vi "hmi_initialize.vi"(4 "dialog_type":T3=enum."one_button", 6 "configuration":T2={"dialog_text"="", "boolean_text_1"="", "boolean_text_2"="", "boolean_text_3"="", "inner_color"=16711680, "outer_color"=6618880, "wait_s"=nan, "error_status"=FALSE, "error_source"="", "error_details"="", "string []"=[], "custom_entry"=FALSE}, 7 "references":T1, 8 "error in (no error)":errorcluster) -> (0 "error out":errorcluster)   [LabVIEW 2015, in "lv-dialog-interfaces.lvlib"]
uses:
  lv-dialog-interfaces.lvlib
  _controls/dialog_type.ctl
  _controls/configuration.ctl
  _controls/hmi_references.ctl
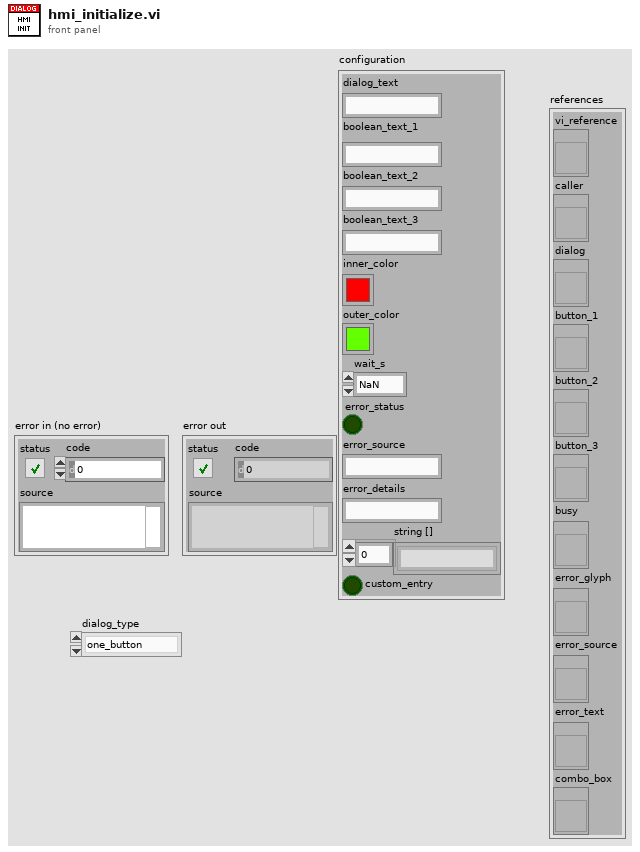
[diagram p1: front panel]
types:
  T1 = typedef "lv-dialog-interfaces.lvlib/hmi_references.ctl" = cluster{"vi_reference":refnum<vi>, "caller":refnum<vi>, "dialog":refnum<vi>, "button_1":refnum<vi>, "button_2":refnum<vi>, "button_3":refnum<vi>, "busy":refnum<vi>, "error_glyph":refnum<vi>, "error_source":refnum<vi>, "error_text":refnum<vi>, "combo_box":refnum<vi>}
  T2 = typedef "lv-dialog-interfaces.lvlib/configuration.ctl" = cluster{"dialog_text":string, "boolean_text_1":string, "boolean_text_2":string, "boolean_text_3":string, "inner_color":u32, "outer_color":u32, "wait_s":dbl, "error_status":bool, "error_source":string, "error_details":string, "string []":string[], "custom_entry":bool}
  T3 = typedef "lv-dialog-interfaces.lvlib/dialog_type.ctl" = enum16{"null", "one_button", "two_button", "three_button", "confirmation", "busy_wait", "error", "busy_wait_embed", "combo_box", "data_entry_string", "data_entry_numeric"}
  T4 = cluster{"max_height":i16, "max_width":i16, "control_height":i16, "control_width":i16}
  T5 = enum8{"Enabled", "Disabled", "Disabled and Grayed Out"}
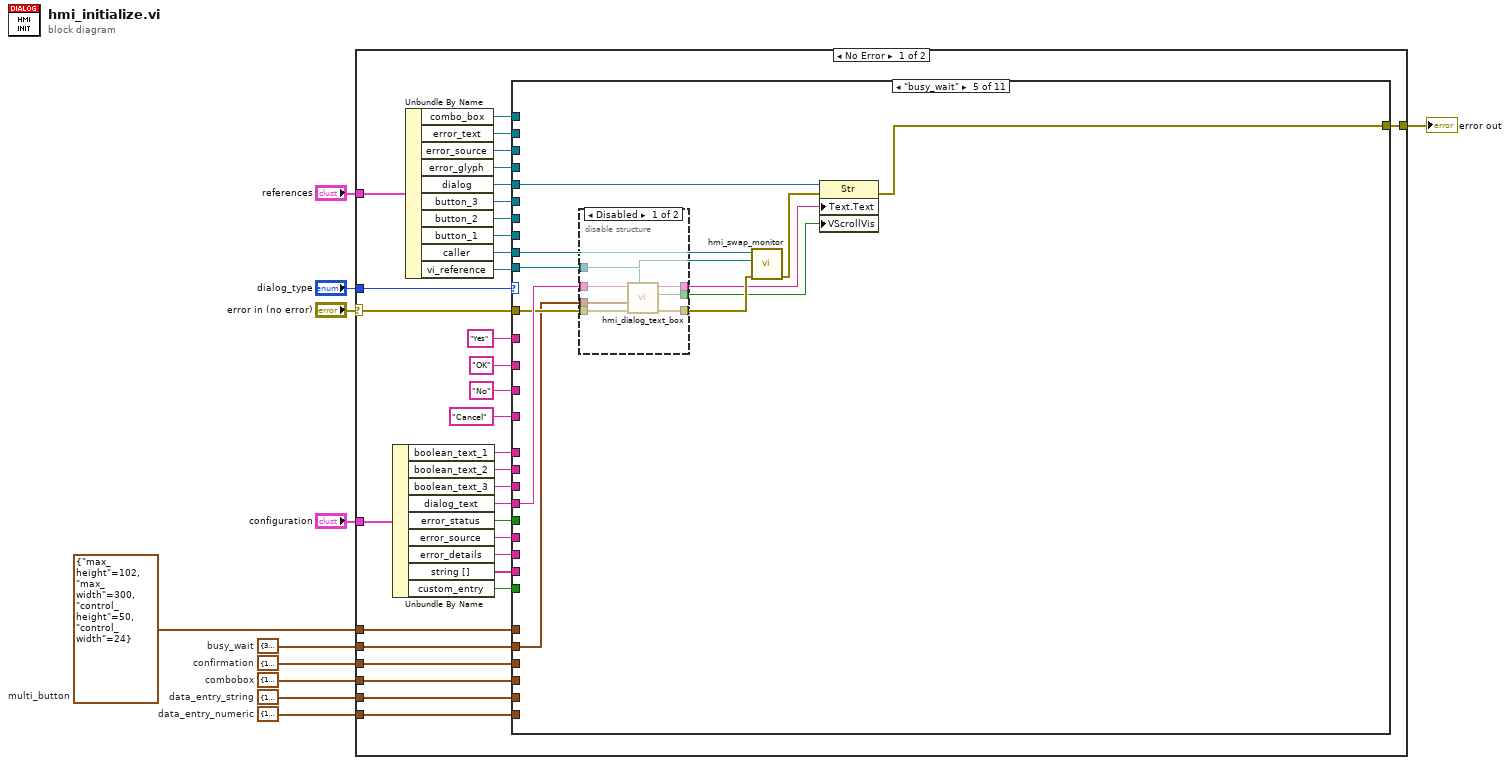
[diagram p0: block diagram]
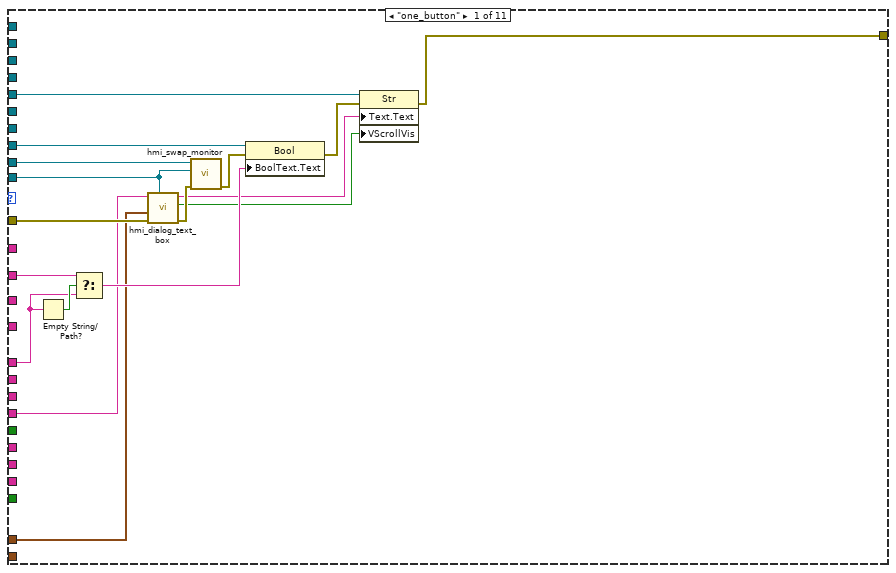
[diagram p2: hidden frame]
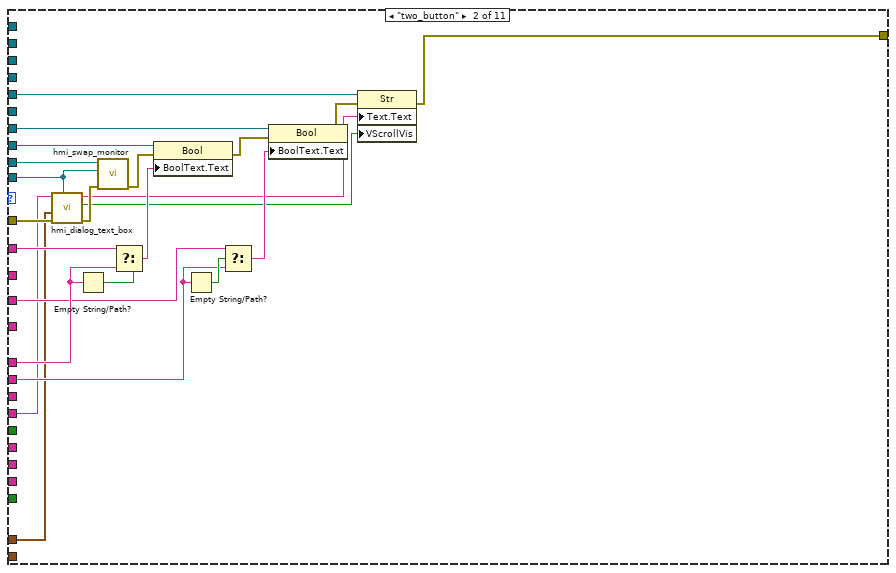
[diagram p3: hidden frame]
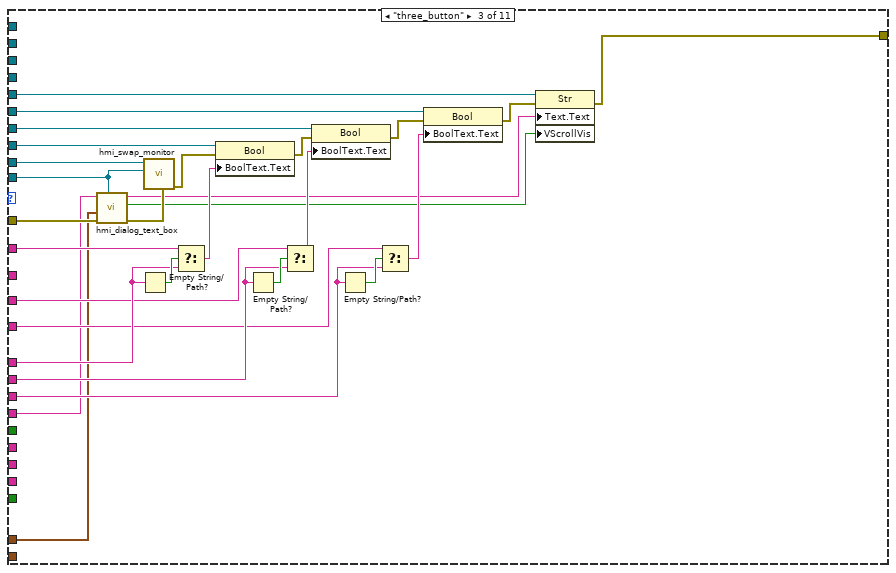
[diagram p4: hidden frame]
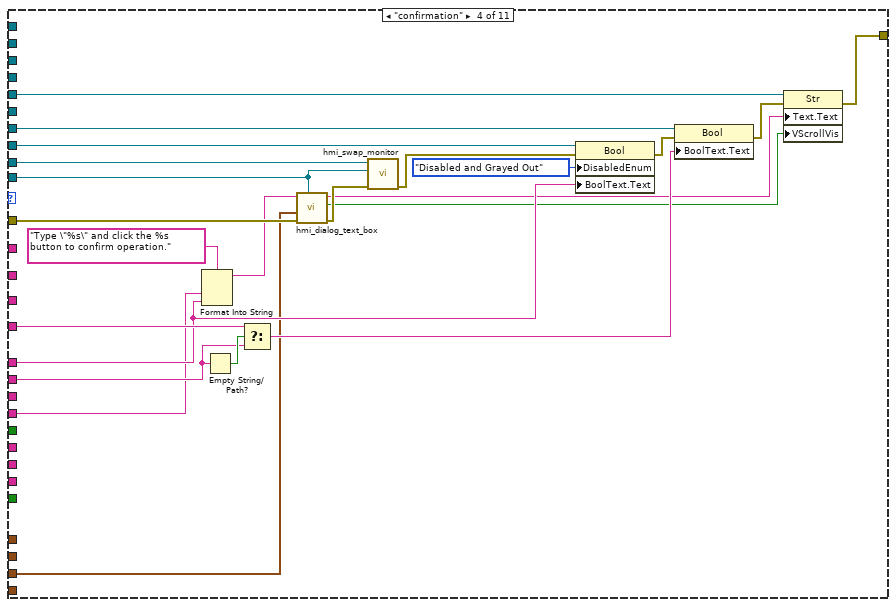
[diagram p5: hidden frame]
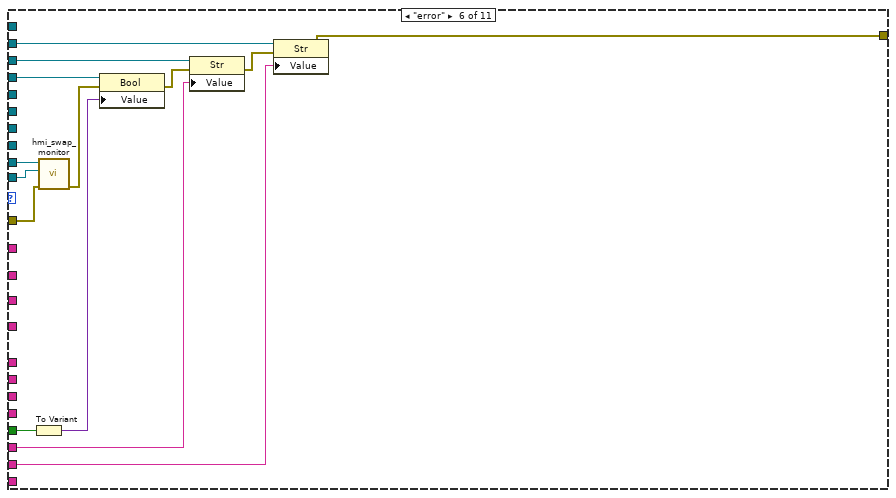
[diagram p7: hidden frame]
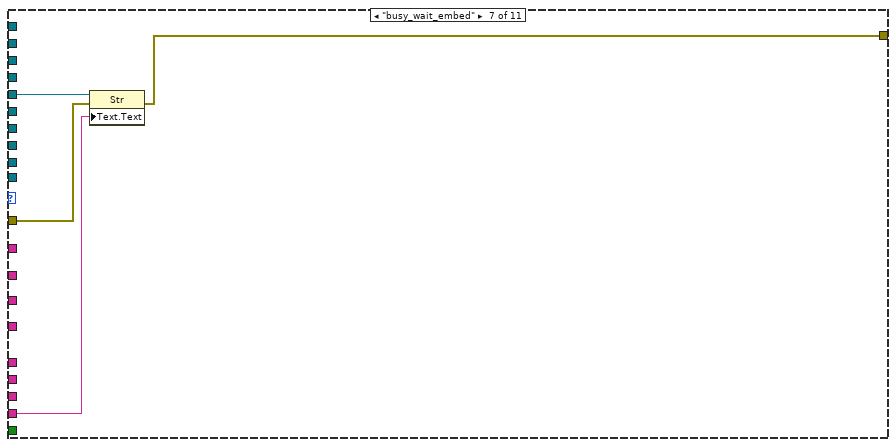
[diagram p8: hidden frame]
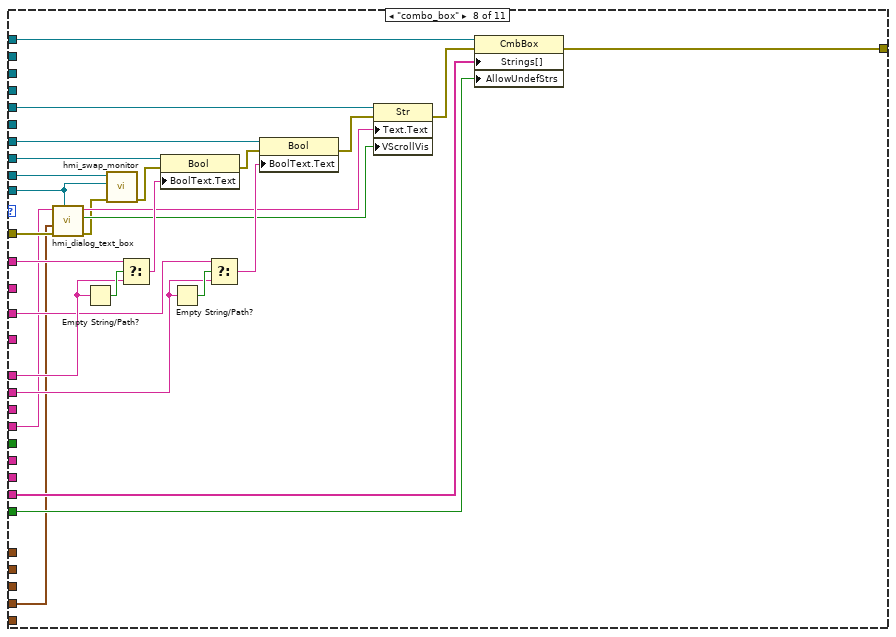
[diagram p9: hidden frame]
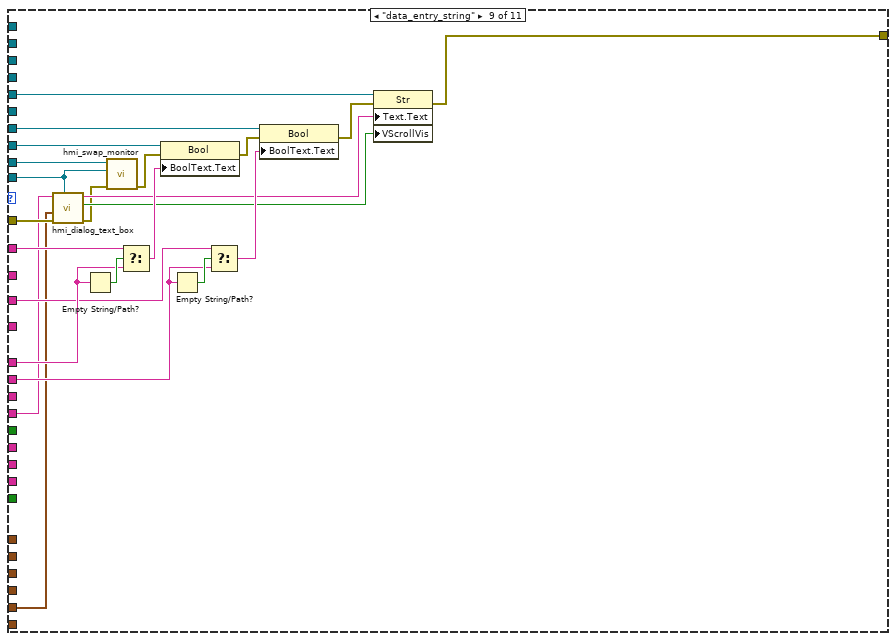
[diagram p10: hidden frame]
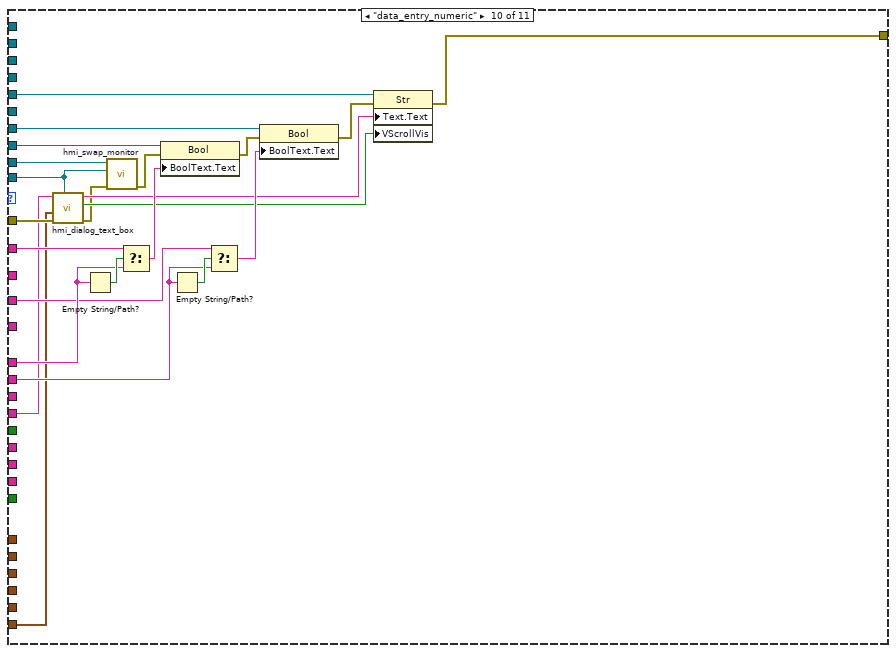
[diagram p11: hidden frame]
diagram:
  w1 = T4 {"max_height"=102, "max_width"=300, "control_height"=50, "control_width"=24}  # data_entry_numeric
  w2 = T4 {"max_height"=102, "max_width"=300, "control_height"=50, "control_width"=24}  # data_entry_string
  w5 = T4 {"max_height"=300, "max_width"=175, "control_height"=175, "control_width"=24}  # busy_wait
  w3 = T4 {"max_height"=102, "max_width"=300, "control_height"=50, "control_width"=24}  # combobox
  w4 = T4 {"max_height"=102, "max_width"=300, "control_height"=50, "control_width"=24}  # confirmation
  w6 = T4 {"max_height"=102, "max_width"=300, "control_height"=50, "control_width"=24}  # multi_button
  n1 = case shown="No Error" "error in (no error)" {
    selector: "error in (no error)" -> [w28 w250]
    tunnel: [w44 w250] -> w10
    tunnel: "dialog_type" -> [w45 _]
    tunnel: "configuration" -> [w39 _]
    tunnel: "references" -> [w43 _]
    tunnel: w6 -> [w17 _]
    tunnel: w5 -> [w16 _]
    tunnel: w4 -> [w15 _]
    tunnel: w3 -> [w14 _]
    tunnel: w2 -> [w13 _]
    tunnel: w1 -> [w12 _]
    frame No Error {
      n2 = Unbundle By Name(w39) -> ("boolean_text_1"=w38:string, "boolean_text_2"=w37:string, "boolean_text_3"=w36:string, "dialog_text"=w35:string, "error_status"=w27:bool, "error_source"=w26:string, "error_details"=w25:string, "string []"=w19:string[], "custom_entry"=w18:bool)
      n3 = Unbundle By Name(w43) -> ("combo_box"=w20:refnum<vi>, "error_text"=w24:refnum<vi>, "error_source"=w23:refnum<vi>, "error_glyph"=w22:refnum<vi>, "dialog"=w42:refnum<vi>, "button_3"=w41:refnum<vi>, "button_2"=w40:refnum<vi>, "button_1"=w34:refnum<vi>, "caller"=w21:refnum<vi>, "vi_reference"=w29:refnum<vi>)
      n4 = case shown="\"busy_wait\"" w45 {
        tunnel: w28 -> [w55 w70 w91 w121 w146 w162 w172 w185 w211 w234 w249]
        tunnel: [w52 w63 w93 w123 w140 w163 w173 w188 w204 w227 w249] -> w44
        tunnel: w42 -> [w53 w67 w94 w133 w141 _ w174 w182 w208 w231 _]
        tunnel: w41 -> [_ _ w114 _ _ _ _ _ _ _ _]
        tunnel: w40 -> [_ w85 w113 w137 _ _ _ w202 w225 w248 _]
        tunnel: w38 -> [w61 w83 w111 w127 _ _ _ w200 w223 w246 _]
        tunnel: w37 -> [_ w81 w108 w135 _ _ _ w198 w221 w244 _]
        tunnel: w36 -> [_ _ w107 _ _ _ _ _ _ _ _]
        tunnel: w35 -> [w47 w69 w89 w117 w147 _ w175 w184 w210 w233 _]
        tunnel: w34 -> [w60 w78 w103 w134 _ _ _ w195 w218 w241 _]
        tunnel: "OK" -> [w58 _ _ _ _ _ _ _ _ _ _]
        tunnel: "Cancel" -> [_ _ w104 w130 _ _ _ _ _ _ _]
        tunnel: "Yes" -> [_ w80 w106 _ _ _ _ w197 w220 w243 _]
        tunnel: "No" -> [_ w79 w105 _ _ _ _ w196 w219 w242 _]
        tunnel: w27 -> [_ _ _ _ _ w168 _ _ _ _ _]
        tunnel: w26 -> [_ _ _ _ _ w167 _ _ _ _ _]
        tunnel: w25 -> [_ _ _ _ _ w166 _ _ _ _ _]
        tunnel: w24 -> [_ _ _ _ _ w169 _ _ _ _ _]
        tunnel: w23 -> [_ _ _ _ _ w170 _ _ _ _ _]
        tunnel: w22 -> [_ _ _ _ _ w171 _ _ _ _ _]
        tunnel: w21 -> [w57 w74 w97 w124 w148 w160 _ w191 w214 w237 _]
        tunnel: w29 -> [w51 w71 w90 w122 w139 w159 _ w186 w212 w235 _]
        tunnel: w20 -> [_ _ _ _ _ _ _ w189 _ _ _]
        tunnel: w19 -> [_ _ _ _ _ _ _ w187 _ _ _]
        tunnel: w17 -> [w46 w68 w87 _ _ _ _ _ _ _ _]
        tunnel: w18 -> [_ _ _ _ _ _ _ w177 _ _ _]
        tunnel: w16 -> [_ _ _ _ w138 _ _ _ _ _ _]
        tunnel: w15 -> [_ _ _ w115 _ _ _ _ _ _ _]
        tunnel: w14 -> [_ _ _ _ _ _ _ w176 _ _ _]
        tunnel: w13 -> [_ _ _ _ _ _ _ _ w203 _ _]
        tunnel: w12 -> [_ _ _ _ _ _ _ _ _ w226 _]
        frame "one_button" {
          n5 = Empty String/Path?(string/path=w61) -> (empty?=w62:bool)
          n6 = Select(t=w58, s=w62, f=w61) -> (s? t:f=w50:string)
          n7 = call "hmi_dialog_text_box.vi"("vi_reference"=w51, "error in (no error)"=w55, "vi_maximums"=w46, "dialog_text in"=w47) -> ("error out"=w54:errorcluster, "enable_scrollbar"=w48:bool, "dialog_text out"=w49:string)  [unwired: 5 in]
          n8 = call "hmi_swap_monitor.vi"("error in (no error)"=w54, "callee_vi_refnum"=w51, "caller_vi_refnum"=w57) -> ("error out"=w56:errorcluster)  [unwired: 8 in]
          n9 = property class="Bool"(reference=w60, error in=w56, "BoolText.Text"=w50) -> (error out=w59:errorcluster)  [unwired: 1 out]
          n10 = property class="Str"(reference=w53, error in=w59, "Text.Text"=w49, "VScrollVis"=w48) -> (error out=w52:errorcluster)  [unwired: 1 out]
        }
        frame "two_button" {
          n11 = call "hmi_dialog_text_box.vi"("vi_reference"=w71, "error in (no error)"=w70, "vi_maximums"=w68, "dialog_text in"=w69) -> ("error out"=w72:errorcluster, "enable_scrollbar"=w65:bool, "dialog_text out"=w66:string)  [unwired: 5 in]
          n12 = Empty String/Path?(string/path=w83) -> (empty?=w84:bool)
          n13 = call "hmi_swap_monitor.vi"("error in (no error)"=w72, "callee_vi_refnum"=w71, "caller_vi_refnum"=w74) -> ("error out"=w73:errorcluster)  [unwired: 8 in]
          n14 = Select(t=w80, s=w84, f=w83) -> (s? t:f=w77:string)
          n15 = property class="Bool"(reference=w78, error in=w73, "BoolText.Text"=w77) -> (error out=w75:errorcluster)  [unwired: 1 out]
          n16 = Empty String/Path?(string/path=w81) -> (empty?=w82:bool)
          n17 = Select(t=w79, s=w82, f=w81) -> (s? t:f=w76:string)
          n18 = property class="Bool"(reference=w85, error in=w75, "BoolText.Text"=w76) -> (error out=w64:errorcluster)  [unwired: 1 out]
          n19 = property class="Str"(reference=w67, error in=w64, "Text.Text"=w66, "VScrollVis"=w65) -> (error out=w63:errorcluster)  [unwired: 1 out]
        }
        frame "three_button" {
          n20 = call "hmi_dialog_text_box.vi"("vi_reference"=w90, "error in (no error)"=w91, "vi_maximums"=w87, "dialog_text in"=w89) -> ("error out"=w92:errorcluster, "enable_scrollbar"=w86:bool, "dialog_text out"=w88:string)  [unwired: 5 in]
          n21 = Empty String/Path?(string/path=w111) -> (empty?=w112:bool)
          n22 = call "hmi_swap_monitor.vi"("error in (no error)"=w92, "callee_vi_refnum"=w90, "caller_vi_refnum"=w97) -> ("error out"=w96:errorcluster)  [unwired: 8 in]
          n23 = Select(t=w106, s=w112, f=w111) -> (s? t:f=w102:string)
          n24 = property class="Bool"(reference=w103, error in=w96, "BoolText.Text"=w102) -> (error out=w99:errorcluster)  [unwired: 1 out]
          n25 = Empty String/Path?(string/path=w108) -> (empty?=w110:bool)
          n26 = Select(t=w105, s=w110, f=w108) -> (s? t:f=w101:string)
          n27 = property class="Bool"(reference=w113, error in=w99, "BoolText.Text"=w101) -> (error out=w98:errorcluster)  [unwired: 1 out]
          n28 = Empty String/Path?(string/path=w107) -> (empty?=w109:bool)
          n29 = Select(t=w104, s=w109, f=w107) -> (s? t:f=w100:string)
          n30 = property class="Bool"(reference=w114, error in=w98, "BoolText.Text"=w100) -> (error out=w95:errorcluster)  [unwired: 1 out]
          n31 = property class="Str"(reference=w94, error in=w95, "Text.Text"=w88, "VScrollVis"=w86) -> (error out=w93:errorcluster)  [unwired: 1 out]
        }
        frame "confirmation" {
          n32 = Format Into String(format string="Type \"%s\" and click the %s button to confirm operation.", w117, w127) -> (resulting string=w116:string)  [unwired: 2 in, 1 out]
          n33 = Empty String/Path?(string/path=w135) -> (empty?=w136:bool)
          n34 = Select(t=w130, s=w136, f=w135) -> (s? t:f=w132:string)
          n35 = call "hmi_dialog_text_box.vi"("vi_reference"=w122, "error in (no error)"=w121, "vi_maximums"=w115, "dialog_text in"=w116) -> ("error out"=w120:errorcluster, "enable_scrollbar"=w119:bool, "dialog_text out"=w118:string)  [unwired: 5 in]
          n36 = call "hmi_swap_monitor.vi"("error in (no error)"=w120, "callee_vi_refnum"=w122, "caller_vi_refnum"=w124) -> ("error out"=w125:errorcluster)  [unwired: 8 in]
          n37 = property class="Bool"(reference=w134, error in=w125, "DisabledEnum"=T5."Disabled and Grayed Out" ("Disabled"), "BoolText.Text"=w127) -> (error out=w131:errorcluster)  [unwired: 1 out]
          n38 = property class="Bool"(reference=w137, error in=w131, "BoolText.Text"=w132) -> (error out=w129:errorcluster)  [unwired: 1 out]
          n39 = property class="Str"(reference=w133, error in=w129, "Text.Text"=w118, "VScrollVis"=w119) -> (error out=w123:errorcluster)  [unwired: 1 out]
        }
        frame "busy_wait" {
          n40 = disable-structure shown="Disabled" {
            disable-tunnel: w147 -> [w155 w157]
            disable-tunnel: w146 -> [w154 w156]
            disable-tunnel: [w153 w156] -> w145
            disable-tunnel: [w152 w157] -> w144
            disable-tunnel: [w151 _] -> w143
            disable-tunnel: w139 -> [w150 _]
            disable-tunnel: w138 -> [w149 _]
            frame Disabled {
              n41 = call "hmi_dialog_text_box.vi"("vi_reference"=w150, "error in (no error)"=w154, "vi_maximums"=w149, "dialog_text in"=w155) -> ("error out"=w153:errorcluster, "enable_scrollbar"=w151:bool, "dialog_text out"=w152:string)  [unwired: 5 in]
            }
            frame Enabled {
            }
          }
          n42 = call "hmi_swap_monitor.vi"("error in (no error)"=w145, "callee_vi_refnum"=w139, "caller_vi_refnum"=w148) -> ("error out"=w142:errorcluster)  [unwired: 8 in]
          n43 = property class="Str"(reference=w141, error in=w142, "Text.Text"=w144, "VScrollVis"=w143) -> (error out=w140:errorcluster)  [unwired: 1 out]
        }
        frame "error" {
          n44 = To Variant(anything=w168) -> (Variant=w158:variant)
          n45 = call "hmi_swap_monitor.vi"("error in (no error)"=w162, "callee_vi_refnum"=w159, "caller_vi_refnum"=w160) -> ("error out"=w161:errorcluster)  [unwired: 8 in]
          n46 = property class="Bool"(reference=w171, error in=w161, "Value"=w158) -> (error out=w165:errorcluster)  [unwired: 1 out]
          n47 = property class="Str"(reference=w170, error in=w165, "Value"=w167) -> (error out=w164:errorcluster)  [unwired: 1 out]
          n48 = property class="Str"(reference=w169, error in=w164, "Value"=w166) -> (error out=w163:errorcluster)  [unwired: 1 out]
        }
        frame "busy_wait_embed" {
          n49 = property class="Str"(reference=w174, error in=w172, "Text.Text"=w175) -> (error out=w173:errorcluster)  [unwired: 1 out]
        }
        frame "combo_box" {
          n50 = call "hmi_dialog_text_box.vi"("vi_reference"=w186, "error in (no error)"=w185, "vi_maximums"=w176, "dialog_text in"=w184) -> ("error out"=w178:errorcluster, "enable_scrollbar"=w179:bool, "dialog_text out"=w180:string)  [unwired: 5 in]
          n51 = Empty String/Path?(string/path=w200) -> (empty?=w201:bool)
          n52 = call "hmi_swap_monitor.vi"("error in (no error)"=w178, "callee_vi_refnum"=w186, "caller_vi_refnum"=w191) -> ("error out"=w190:errorcluster)  [unwired: 8 in]
          n53 = Select(t=w197, s=w201, f=w200) -> (s? t:f=w194:string)
          n54 = property class="Bool"(reference=w195, error in=w190, "BoolText.Text"=w194) -> (error out=w192:errorcluster)  [unwired: 1 out]
          n55 = Empty String/Path?(string/path=w198) -> (empty?=w199:bool)
          n56 = Select(t=w196, s=w199, f=w198) -> (s? t:f=w193:string)
          n57 = property class="Bool"(reference=w202, error in=w192, "BoolText.Text"=w193) -> (error out=w183:errorcluster)  [unwired: 1 out]
          n58 = property class="Str"(reference=w182, error in=w183, "Text.Text"=w180, "VScrollVis"=w179) -> (error out=w181:errorcluster)  [unwired: 1 out]
          n59 = property class="CmbBox"(reference=w189, error in=w181, "Strings[]"=w187, "AllowUndefStrs"=w177) -> (error out=w188:errorcluster)  [unwired: 1 out]
        }
        frame "data_entry_string" {
          n60 = call "hmi_dialog_text_box.vi"("vi_reference"=w212, "error in (no error)"=w211, "vi_maximums"=w203, "dialog_text in"=w210) -> ("error out"=w205:errorcluster, "enable_scrollbar"=w206:bool, "dialog_text out"=w207:string)  [unwired: 5 in]
          n61 = Empty String/Path?(string/path=w223) -> (empty?=w224:bool)
          n62 = call "hmi_swap_monitor.vi"("error in (no error)"=w205, "callee_vi_refnum"=w212, "caller_vi_refnum"=w214) -> ("error out"=w213:errorcluster)  [unwired: 8 in]
          n63 = Select(t=w220, s=w224, f=w223) -> (s? t:f=w217:string)
          n64 = property class="Bool"(reference=w218, error in=w213, "BoolText.Text"=w217) -> (error out=w215:errorcluster)  [unwired: 1 out]
          n65 = Empty String/Path?(string/path=w221) -> (empty?=w222:bool)
          n66 = Select(t=w219, s=w222, f=w221) -> (s? t:f=w216:string)
          n67 = property class="Bool"(reference=w225, error in=w215, "BoolText.Text"=w216) -> (error out=w209:errorcluster)  [unwired: 1 out]
          n68 = property class="Str"(reference=w208, error in=w209, "Text.Text"=w207, "VScrollVis"=w206) -> (error out=w204:errorcluster)  [unwired: 1 out]
        }
        frame "data_entry_numeric" {
          n69 = call "hmi_dialog_text_box.vi"("vi_reference"=w235, "error in (no error)"=w234, "vi_maximums"=w226, "dialog_text in"=w233) -> ("error out"=w228:errorcluster, "enable_scrollbar"=w229:bool, "dialog_text out"=w230:string)  [unwired: 5 in]
          n70 = Empty String/Path?(string/path=w246) -> (empty?=w247:bool)
          n71 = call "hmi_swap_monitor.vi"("error in (no error)"=w228, "callee_vi_refnum"=w235, "caller_vi_refnum"=w237) -> ("error out"=w236:errorcluster)  [unwired: 8 in]
          n72 = Select(t=w243, s=w247, f=w246) -> (s? t:f=w240:string)
          n73 = property class="Bool"(reference=w241, error in=w236, "BoolText.Text"=w240) -> (error out=w238:errorcluster)  [unwired: 1 out]
          n74 = Empty String/Path?(string/path=w244) -> (empty?=w245:bool)
          n75 = Select(t=w242, s=w245, f=w244) -> (s? t:f=w239:string)
          n76 = property class="Bool"(reference=w248, error in=w238, "BoolText.Text"=w239) -> (error out=w232:errorcluster)  [unwired: 1 out]
          n77 = property class="Str"(reference=w231, error in=w232, "Text.Text"=w230, "VScrollVis"=w229) -> (error out=w227:errorcluster)  [unwired: 1 out]
        }
        frame Default {
        }
      }
    }
    frame Error {
    }
  }
  "error out" <- w10
